vi "Excel To PDF.vi"(7 "Report Type":T1(ring)=enum."Excel", 8 "error in":errorcluster, 10 "PDF Filename":path=path "Appended Report.pdf", 11 "Excel Path":path=path "Appended Report.xls") -> (0 "error out":errorcluster)   [LabVIEW 2013]
uses:
  <vilib>/Utility/NIReport.llb/NI_report.lvclass
  <vilib>/Utility/NIReport.llb/Word/NI_Word.lvclass
  <vilib>/Utility/NIReport.llb/Excel/NI_Excel.lvclass
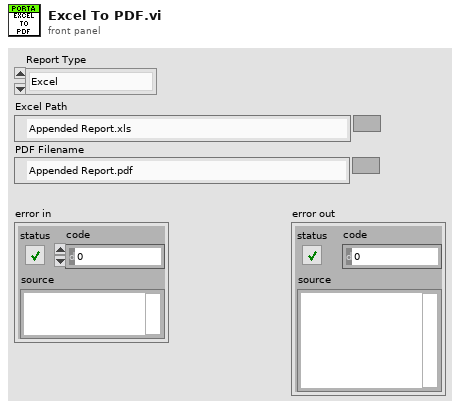
[diagram p1: front panel]
types:
  T1 = enum16{"Standard Report", "HTML", "Word", "Excel"}
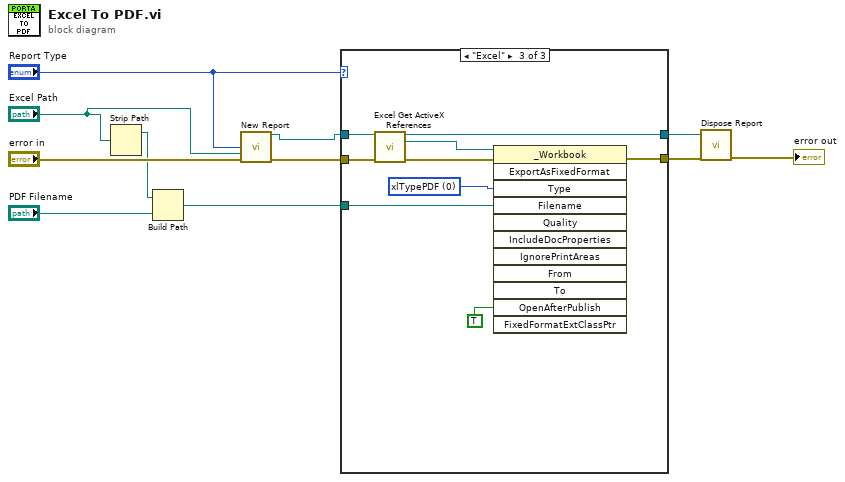
[diagram p0: block diagram]
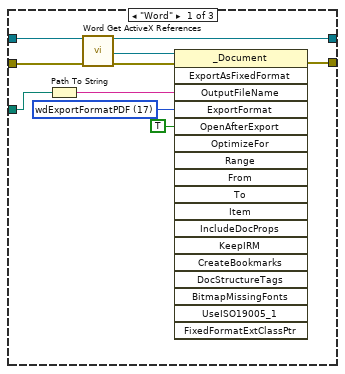
[diagram p2: hidden frame]
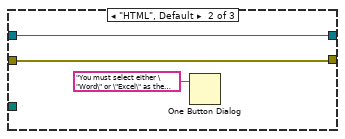
[diagram p3: hidden frame]
diagram:
  n1 = Strip Path(path="Excel Path") -> (stripped path=w2:path)  [unwired: 1 out]
  n2 = Build Path(base path=w2, name or relative path="PDF Filename") -> (appended path=w7:path)
  n3 = call <vilib>:"New Report.vi"("report type"="Report Type", "template (empty)"="Excel Path", "error in (no error)"="error in") -> ("report out"=w3:refnum<class "NI_report.lvclass">, "error out"=w10:errorcluster)  [unwired: 11 in]
  n4 = case shown="\"Excel\"" "Report Type" {
    tunnel: w3 -> [w21 w24 w33]
    tunnel: w7 -> [w18 _ w31]
    tunnel: [w20 w24 w29] -> w8
    tunnel: w10 -> [w15 w22 w28]
    tunnel: [w13 w22 w26] -> w11
    frame "Word" {
      w16 = 17 items=["wdExportFormatPDF"=17, "wdExportFormatXPS"=18] ("ExportFormat")
      n5 = Path To String(path=w18) -> (string=w17:string)
      n6 = call <vilib>:"Word Get ActiveX References.vi"("report in"=w21, "error in (no error)"=w15) -> ("report out"=w20:refnum<class "NI_report.lvclass">, "Word._Document"=w19:refnum<k7>, "error out"=w14:errorcluster)  [unwired: 7 in, 4 out]
      n7 = invoke class="_Document" method="ExportAsFixedFormat"(reference=w19, error in=w14, "OutputFileName"=w17, "ExportFormat"=w16, "OpenAfterExport"=TRUE) -> (error out=w13:errorcluster)  [unwired: 13 in, 17 out]
    }
    frame "HTML", Default {
      n8 = One Button Dialog(message="You must select either \"Word\" or \"Excel\" as the Report Type.") -> ()  [unwired: 1 in, 1 out]
    }
    frame "Excel" {
      w32 = 0 items=["xlTypePDF", "xlTypeXPS"] ("Type")
      n9 = call <vilib>:"Excel Get ActiveX References.vi"("report in"=w33, "error in (no error)"=w28) -> ("report out"=w29:refnum<class "NI_report.lvclass">, "Excel._Workbook"=w25:refnum<k7>, "error out"=w27:errorcluster)  [unwired: 7 in, 4 out]
      n10 = invoke class="_Workbook" method="ExportAsFixedFormat"(reference=w25, error in=w27, "Type"=w32, "Filename"=w31, "OpenAfterPublish"=TRUE) -> (error out=w26:errorcluster)  [unwired: 7 in, 11 out]
    }
  }
  n11 = call-dynamic "Dispose Report.vi"("report in"=w8, "error in (no error)"=w11) -> ("error out"=→"error out":errorcluster)  [unwired: 13 in]
